vi "Configure Chan Characteristics.vi"(0 "VISA Resource Name":refnum<visa-resource-name>, 5 "Channel Name (\"Channel 1\")":string(combo)="CHAN1", 7 "Input Impedance (1.0 mega ohm)":string(combo)="ONEMEG", 9 "Max Input Frequency (20.0E+6 Hz)":string(combo)="1", 11 "error in (no error)":errorcluster {"code" format="%.0x"}) -> (4 "VISA Resource Name Out":refnum<visa-resource-name>, 15 "error out":errorcluster {"code" format="%.0x"})   [LabVIEW 2011, in "Agilent 546XX Series.lvlib"]
doc: "This VI configures the properties that control the electrical characteristics of the channel. These properties are the input impedance and the bandwidth.\n\nNote: This VI has effect only on analog channels. If you want to configure digital channel, use VI ag546xx Configure Digital Channel instead."
uses:
  Agilent 546XX Series.lvlib
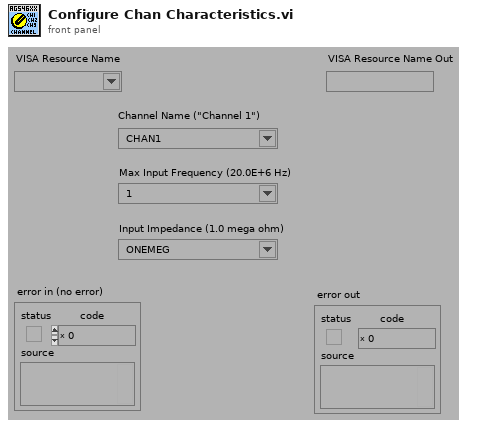
[diagram p1: front panel]
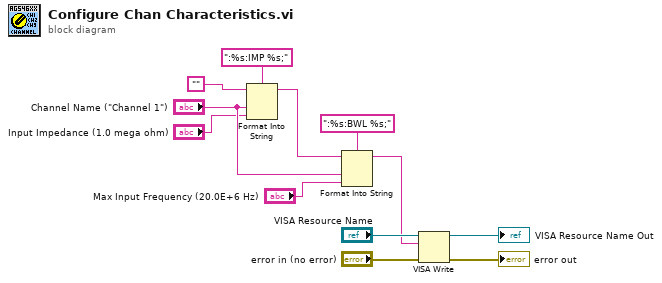
[diagram p0: block diagram]
diagram:
  n1 = Format Into String(format string=":%s:IMP %s;", initial string="", "Channel Name (\"Channel 1\")", "Input Impedance (1.0 mega ohm)") -> (resulting string=w1:string)  [unwired: 1 in, 1 out]
  n2 = Format Into String(format string=":%s:BWL %s;", initial string=w1, "Channel Name (\"Channel 1\")", "Max Input Frequency (20.0E+6 Hz)") -> (resulting string=w2:string)  [unwired: 1 in, 1 out]
  n3 = VISA Write(VISA resource name="VISA Resource Name", write buffer=w2, error in (no error)="error in (no error)") -> (VISA resource name out=→"VISA Resource Name Out":refnum<visa-resource-name>, error out=→"error out":errorcluster)  [unwired: 1 out]
